vi "OverlayRoi.vi"(6 "Colors":u32[](array[colorbox])=[6618880], 7 "GroupName":string, 8 "error in":errorcluster, 9 "Point Symbol":u32[][](array[colorbox])=[[16777216, 16777216, 16777216, 0, 16777216, 16777216, 16777216], [16777216, 16777216, 16777216, 0, 16777216, 16777216, 16777216], [16777216, 16777216, 16777216, 0, 16777216, 16777216, 16777216], [0, 0, 0, 16777216, 0, 0, 0], [16777216, 16777216, 16777216, 0, 16777216, 16777216, 16777216], [16777216, 16777216, 16777216, 0, 16777216, 16777216, 16777216], [16777216, 16777216, 16777216, 0, 16777216, 16777216, 16777216]], 10 "ROI Descriptor":T1 {"Contours"."Type" items=["No Selection", "Point", "Line", "Rectangle", "Oval", "Polygon", "Freehand Region", "Annulus", "Unused2", "Unused3", "Broken Line", "Freehand Line", "Rotated Rectangle"]}, 11 "Image Reference In":T2) -> (0 "error out":errorcluster, 3 "Image Reference Out":T2)   [LabVIEW 2024, in "OpenLvVision_Overlays.lvlib"]
doc: "Overlays an ROI (region of interest) into an image."
uses:
  OpenLvVision_Overlays.lvlib
  <vilib>/OpenLvVision/OpenLvVision_Image/Management/TypeDef/OLV Image.ctl
  <vilib>/OpenLvVision/OpenLvVision_Image/Management/OLV Management.lvlib
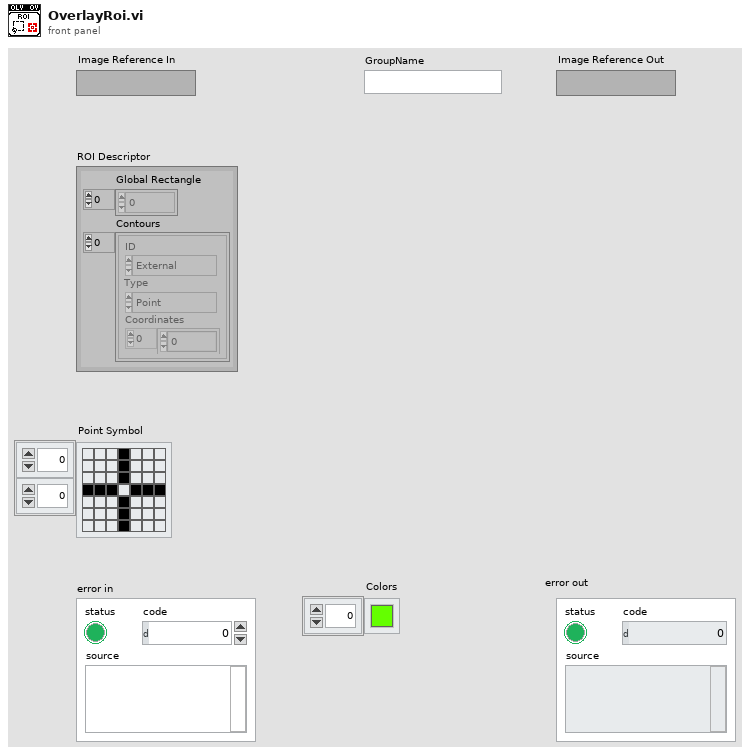
[diagram p1: front panel]
types:
  T1 = typedef "ROI Descriptor" = cluster{"Global Rectangle":i32[], "Contours":cluster{"ID":enum32{"External", "Internal"}, "Type":u32, "Coordinates":i32[]}[]}
  T2 = typedef "OLV OpenLvVision_Image.lvlib/OLV Management.lvlib/OLV Image.ctl" = refnum<image>
  T3 = typedef "IMAQ Image.ctl" = refnum<image>
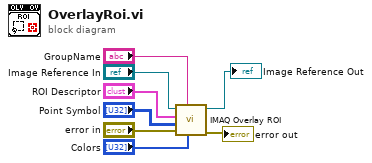
[diagram p0: block diagram]
diagram:
  n1 = call "IMAQ Overlay ROI"("Colors (Green)"="Colors", "Group"="GroupName", "error in (no error)"="error in", "Point Symbol"="Point Symbol", "ROI Descriptor"="ROI Descriptor", "Image"="Image Reference In") -> ("error out"=→"error out":errorcluster, "Image Out"=→"Image Reference Out":T3)  [unwired: 4 in]
